vi "Questionable Status Query.vi"(0 "VISA resource name":refnum<visa-resource-name>, 11 "error in (no error)":errorcluster) -> (4 "VISA resource name out":refnum<visa-resource-name>, 6 "Questionable Status":T1, 15 "error out":errorcluster)   [LabVIEW 2020, in "NH Research Regenerative Test Series.lvlib"]
doc: "Returns the integer data explaining the questionable status monitored in the instrument.\n\nThe Questionable Register consists of the following 16 bits:\n\nBit 0: Reserved\nBit 1: Reserved\nBit 2: Reserved \nBit 3: Reserved\nBit 4: Reserved\nBit 5: Reserved \nBit 6: Reserved\nBit 7: Reserved\nBit 8: Calibration checksum error\nBit 9: Firmware checksum error\nBit 10: Program executing from flash\nBit 11: Installed flash is not detected or incorrect\nBit 12: Reserved\nBit 13: Reserved\nBit 14: Reserved"
uses:
  NH Research Regenerative Test Series.lvlib
panel:
  # "Bit 0:  Reserved\nBit 1:  Reserved\nBit 2:  Reserved\t\nBit 3:  Reserved\nBit 4:\t\tReserved\nBit 5:  Reserved\t\nBit 6:  Reserved\nBit 7:  Reserved\nBit 8:  Calibration checksum error\nBit 9:  Firmware checksum error\nBit 10:  Program executing from flash\nBit 11:  Installed flash is not detected or incorrect\nBit 12:  Reserved\nBit 13:  Reserved\nBit 14:  Reserved"
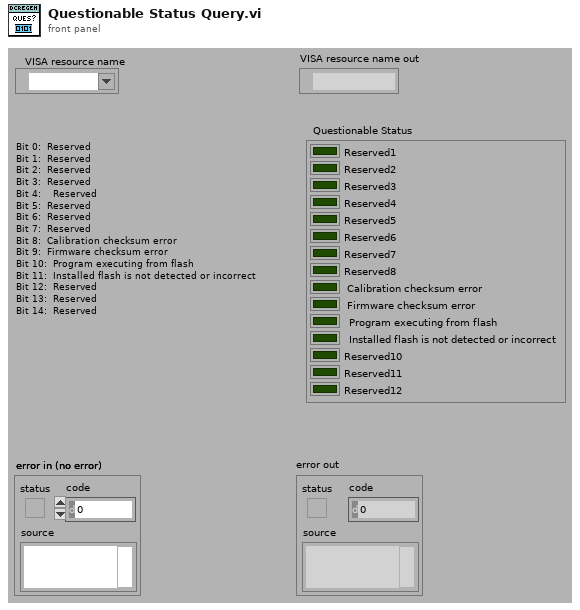
[diagram p1: front panel]
types:
  T1 = cluster{"Reserved1":bool, "Reserved2":bool, "Reserved3":bool, "Reserved4":bool, "Reserved5":bool, "Reserved6":bool, "Reserved7":bool, "Reserved8":bool, "Calibration checksum error":bool, "Firmware checksum error":bool, "Program executing from flash":bool, "Installed flash is not detected or incorrect":bool, "Reserved10":bool, "Reserved11":bool, "Reserved12":bool}
  T2 = cluster{"Operation Complete":bool, "Not Used":bool, "Query Error":bool, "Device Error":bool, "Message Available":bool, "Command Error":bool, "Not Used":bool, "Power On":bool, "Operation Complete 2":bool, "Not Used 2":bool, "Query Error 2":bool, "Device Error 2":bool, "Message Available 2":bool, "Command Error 2":bool, "Not Used 3":bool}
  T3 = cluster{"Boolean array[0]":bool, "Boolean array[1]":bool, "Boolean array[2]":bool, "Boolean array[3]":bool, "Boolean array[4]":bool, "Boolean array[5]":bool, "Boolean array[6]":bool, "Boolean array[7]":bool, "Boolean array[8]":bool, "Boolean array[9]":bool, "Boolean array[10]":bool, "Boolean array[11]":bool, "Boolean array[12]":bool, "Boolean array[13]":bool, "Boolean array[14]":bool}
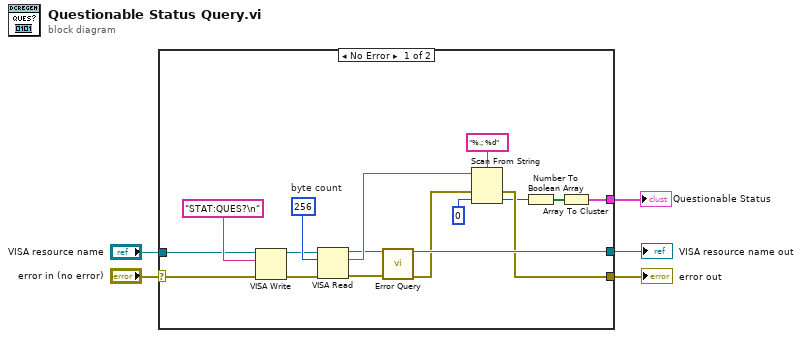
[diagram p0: block diagram]
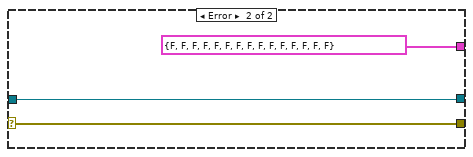
[diagram p2: hidden frame]
diagram:
  n1 = case shown="No Error" "error in (no error)" {
    selector: "error in (no error)" -> [w15 w25]
    tunnel: [w10 w25] -> w5
    tunnel: [w14 w24] -> w4
    tunnel: "VISA resource name" -> [w16 w24]
    tunnel: [w7 T2 {"Operation Complete"=FALSE, "Not Used"=FALSE, "Query Error"=FALSE, "Device Error"=FALSE, "Message Available"=FALSE, "Command Error"=FALSE, "Not Used"=FALSE, "Power On"=FALSE, "Operation Complete 2"=FALSE, "Not Used 2"=FALSE, "Query Error 2"=FALSE, "Device Error 2"=FALSE, "Message Available 2"=FALSE, "Command Error 2"=FALSE, "Not Used 3"=FALSE} ("Operation Status")] -> w1
    frame No Error {
      w21 = u32 256  # byte count
      n2 = VISA Write(VISA resource name=w16, write buffer="STAT:QUES?\n" ("Command to Send (empty)"), error in (no error)=w15) -> (VISA resource name out=w19:refnum<visa-resource-name>, error out=w18:errorcluster)  [unwired: 1 out]
      n3 = VISA Read(VISA resource name=w19, byte count=w21, error in (no error)=w18) -> (VISA resource name out=w13:refnum<visa-resource-name>, read buffer=w20:string, error out=w12:errorcluster)  [unwired: 1 out]
      n4 = call "Error Query.vi"("VISA resource name"=w13, "error in (no error)"=w12) -> ("VISA resource name out"=w14:refnum<visa-resource-name>, "error out"=w11:errorcluster)  [unwired: 10 in, 2 out]
      n5 = Scan From String(format string="%.; %d" ("Format String"), input string=w20, error in=w11, default 1=u16 0 ("default value 1")) -> (error out=w10:errorcluster, output 1=w6:u16)  [unwired: 1 in, 2 out]
      n6 = Number To Boolean Array(number=w6) -> (Boolean array=w9:bool[])
      n7 = Array To Cluster(array=w9) -> (cluster=w7:T3)
    }
    frame Error {
    }
  }
  "error out" <- w5
  "VISA resource name out" <- w4
  "Questionable Status" <- w1
